vi "Read serializeWF_ 2.vi"(8 "error in (no error)":errorcluster, 11 "PAS Cell Data in":refnum<class "PAS Cell Data.lvclass">) -> (0 "error out":errorcluster, 2 "serializeWF?":bool, 3 "PAS Cell Data out":refnum<class "PAS Cell Data.lvclass">)   [LabVIEW 2014, in "PAS Library.lvlib" / "PAS Cell Data.lvclass"]
uses:
  PAS Cell Data.lvclass
  PAS Cell Data.lvclass/PAS Cell Data.ctl
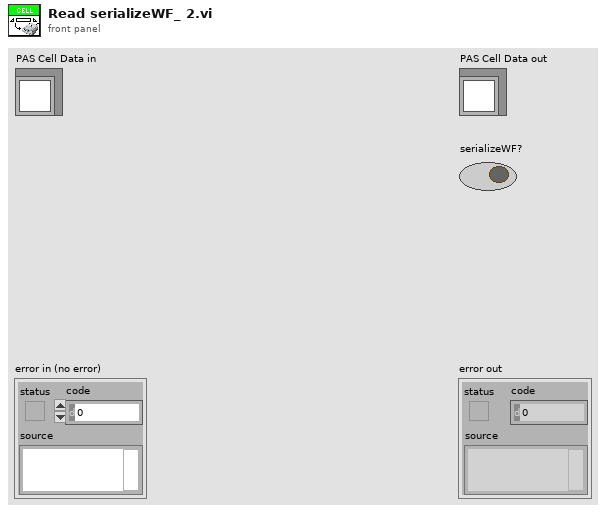
[diagram p1: front panel]
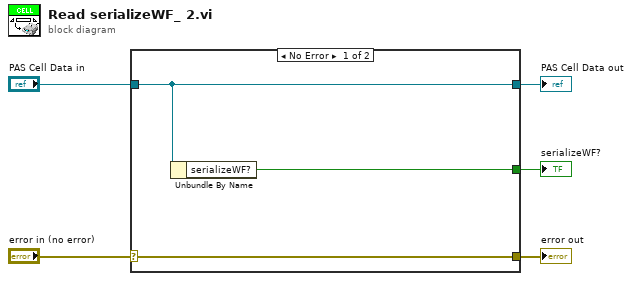
[diagram p0: block diagram]
diagram:
  n1 = case shown="No Error" "error in (no error)" {
    selector: "error in (no error)" -> [w8 w9]
    tunnel: [w8 w9] -> w4
    tunnel: [w7 w10] -> w2
    tunnel: "PAS Cell Data in" -> [w7 w10]
    tunnel: [w6 _] -> w1
    frame No Error {
      n2 = Unbundle By Name(w7) -> ("serializeWF?"=w6:bool)
    }
    frame Error {
    }
  }
  "error out" <- w4
  "PAS Cell Data out" <- w2
  "serializeWF?" <- w1
